vi "Scale_m_x_plus_b.vi"(5 "b":dbl, 7 "m":dbl, 11 "Signal":dbl) -> (3 "Scaled Signal":dbl)   [LabVIEW 2018]
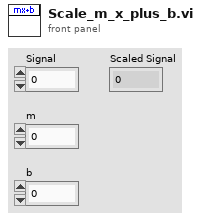
[diagram p1: front panel]
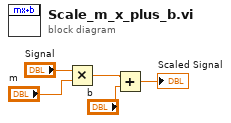
[diagram p0: block diagram]
diagram:
  n1 = Multiply(x="Signal", y="m") -> (x*y=w1:dbl)
  n2 = Add(x=w1, y="b") -> (x+y=→"Scaled Signal":dbl)
